vi "From Pythonic - Float.vi"(4 "Pythonic Value":string) -> (1 "Float":dbl)   [LabVIEW 2012, in "OPI.lvclass"]
doc: "Convert pythonic values into LabVIEW data. This method can be helpfull to convert elements of tuples or dictionaries.\n\nReturn a float - LabVIEW Double representation."
uses:
  OPI.lvclass
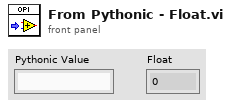
[diagram p1: front panel]
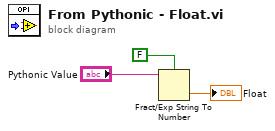
[diagram p0: block diagram]
diagram:
  n1 = Fract/Exp String To Number(use system decimal point (T)=FALSE, string="Pythonic Value") -> (number=→"Float":dbl)  [unwired: 2 in, 1 out]
